vi "startScriptRunList.vi"(8 "error in (no error)":errorcluster, 11 "ExperimentRunner in":refnum<class "ExperimentRunner.lvclass">) -> (0 "error out":errorcluster, 3 "ExperimentRunner out":refnum<class "ExperimentRunner.lvclass">)   [LabVIEW 2009]
uses:
  Tools/Filing/FileSystem/FileSystem.lvclass
  ExperimentRunner.lvclass
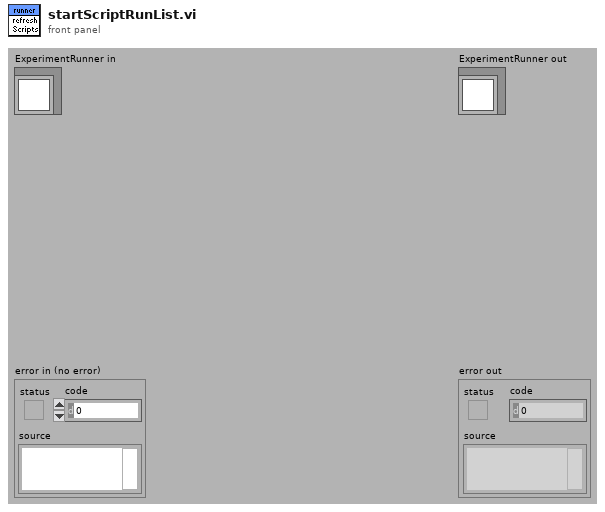
[diagram p1: front panel]
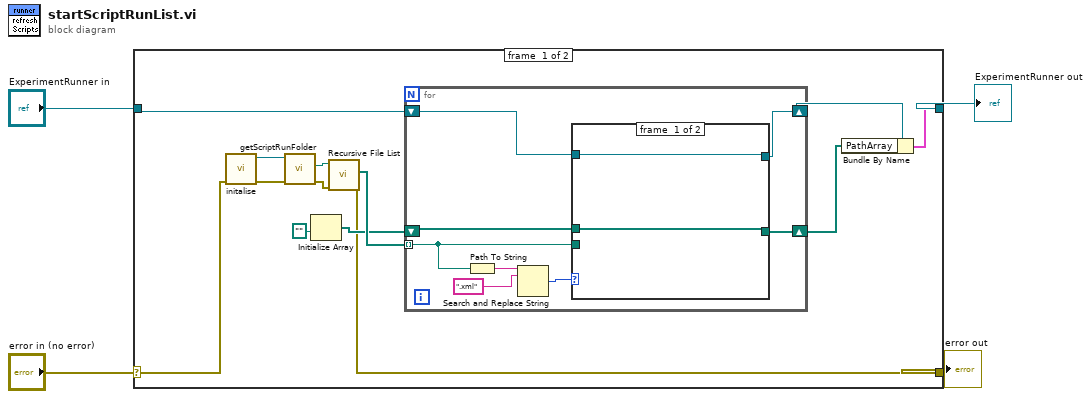
[diagram p0: block diagram]
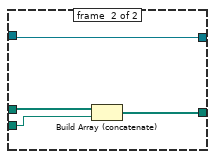
[diagram p2: hidden frame]
diagram:
  n1 = case shown="No Error" "error in (no error)" {
    selector: "error in (no error)" -> [w15 w33]
    tunnel: [w6 w33] -> w3
    tunnel: [w8 w32] -> w1
    tunnel: "ExperimentRunner in" -> [w13 w32]
    frame #0 {
      n2 = call "initalise.vi"("error in (no error)"=w15) -> ("error out"=w16:errorcluster, "FileSystem out"=w17:refnum<class "FileSystem.lvclass">)  [unwired: 9 in]
      n3 = call "getScriptRunFolder.vi"("error in (no error)"=w16, "FileSystem.lvclass in"=w17) -> ("error out"=w5:errorcluster, "ScriptRunFolder"=w14:path)  [unwired: 7 in, 1 out]
      n4 = Initialize Array(path "") -> (w11:path[])  [unwired: 1 in]
      n5 = call <vilib>:"Recursive File List.vi"("error in (no error)"=w5, "Folder Path"=w14) -> ("error out"=w6:errorcluster, "All Files in Dir"=w12:path[])  [unwired: 5 in, 3 out]
      n6 = for {
        tunnel: w12 -> [w21] mode=indexing
        shift-right: [w20] -> w7
        shift-left: w11 -> [w22]
        shift-right: [w18] -> w9
        shift-left: w13 -> [w19]
        n7 = Path To String(path=w21) -> (string=w25:string)
        n8 = Search and Replace String(input string=w25, search string=".xml") -> (number of replacements=w23:i32)  [unwired: 6 in, 3 out]
        n9 = case shown="1, Default" w23 {
          tunnel: w22 -> [w27 w31]
          tunnel: w21 -> [_ w28]
          tunnel: [w27 w30] -> w20
          tunnel: w19 -> [w26 w29]
          tunnel: [w26 w29] -> w18
          frame #0 {
          }
          frame #1 {
            n10 = Build Array (concatenate)(w31, w28) -> (w30:path[])
          }
        }
      }
      n11 = Bundle By Name(cluster=w9, "PathArray"=w7) -> (w8:cluster{})
    }
    frame #1 {
    }
  }
  "error out" <- w3
  "ExperimentRunner out" <- w1
